vi "Charger_Address_Array.vi"(5 "N Positions (6)":i32=6, 6 "error in":errorcluster, 9 "Charger COM Port":refnum<visa-resource-name>="COM17") -> (0 "error out":errorcluster, 2 "Charger":T1[](array[typedef]) {"setpoint" min=0.0 max=20000.0 step=100.0; "position" min=0 max=5 step=1}, 3 "Charger COM dup":refnum<visa-resource-name>="COM17")   [LabVIEW 2020]
uses:
  Drivers/Charger Test Set/Charger_Input Control.ctl
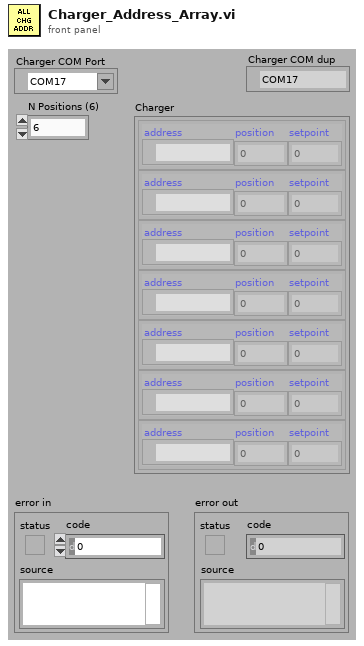
[diagram p1: front panel]
types:
  T1 = typedef "Charger_Input Control.ctl" = cluster{"address":refnum<visa-resource-name>, "position":i32, "setpoint":dbl}
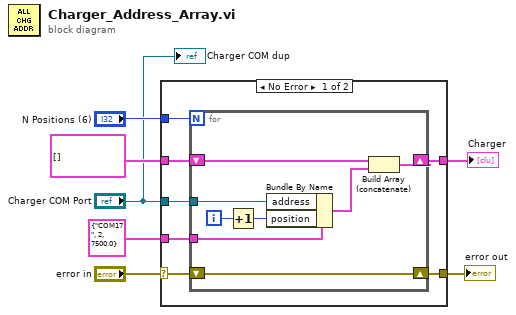
[diagram p0: block diagram]
diagram:
  n1 = case shown="No Error" "error in" {
    selector: "error in" -> [w13 w24]
    tunnel: [w14 w24] -> w7
    tunnel: T1 {"address"="COM17", "position"=2, "setpoint"=7500.0} ("Charger") -> [w12 _]
    tunnel: T1[] [] -> [w11 w23]
    tunnel: [w10 w23] -> w3
    tunnel: "Charger COM Port" -> [w9 _]
    tunnel: "N Positions (6)" -> [w8 _]
    frame No Error {
      n2 = for {
        N: w8 -> [_]
        shift-right: [w17] -> w14
        shift-left: w13 -> [w17]
        shift-right: [w21] -> w10
        shift-left: w11 -> [w22]
        tunnel: w12 -> [w20]
        tunnel: w9 -> [w16]
        i -> [w19]
        n3 = Increment(x=w19) -> (x+1=w15:i32)
        n4 = Bundle By Name(cluster=w20, "address"=w16, "position"=w15) -> (w18:T1)
        n5 = Build Array (concatenate)(w22, w18) -> (w21:T1[])
      }
    }
    frame Error {
    }
  }
  "error out" <- w7
  "Charger" <- w3
  "Charger COM dup" <- "Charger COM Port"
